vi "Subset Plugin State Data.vi"(8 "error in (no error)":errorcluster, 9 "plugin index":i32, 10 "all state data":T1[](array[typedef]) {"period" format="%d us"; "duration" format="%d us"}, 11 "Framework Status in":refnum<class "Framework Status.lvclass">) -> (0 "error out":errorcluster, 1 "groups state data":T1[](array[typedef]) {"period" format="%d us"; "duration" format="%d us"}, 2 "plugin state data":T1 {"period" format="%d us"; "duration" format="%d us"}, 3 "Framework Status out":refnum<class "Framework Status.lvclass">)   [LabVIEW 2019, in "DSF Core.lvlib" / "Framework Status.lvclass"]
uses:
  Framework Status.lvclass
  Status/Status Data.ctl
  Framework Status.lvclass/Framework Status.ctl
  Status/Status Pointer.lvclass
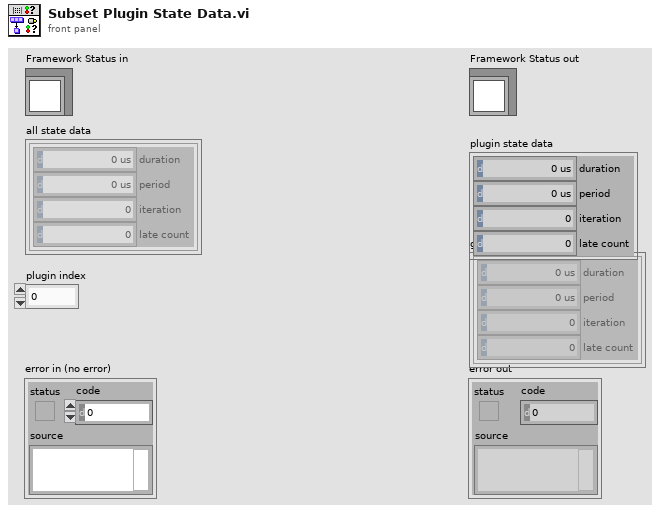
[diagram p1: front panel]
types:
  T1 = typedef "DSF Core.lvlib/Status Pointer.lvclass/Status Data.ctl" = cluster{"duration":u64, "period":u64, "iteration":u64, "late count":u64}
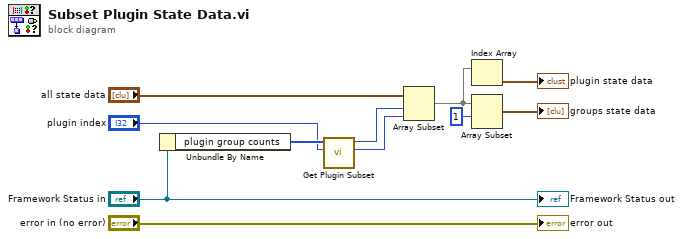
[diagram p0: block diagram]
diagram:
  n1 = Unbundle By Name("Framework Status in") -> ("plugin group counts"=w4:u8[])
  n2 = call "Get Plugin Subset.vi"("plugin index"="plugin index", "plugin group counts"=w4) -> ("length"=w1:u8, "index"=w2:i32)  [unwired: 8 in]
  n3 = Array Subset(array="all state data", index=w2, length=w1) -> (w7:T1[])
  n4 = Index Array(array=w7) -> (element=→"plugin state data":T1)  [unwired: 1 in]
  n5 = Array Subset(array=w7, index=1) -> (→"groups state data":T1[])  [unwired: 1 in]
  "error out" <- "error in (no error)"
  "Framework Status out" <- "Framework Status in"
